vi "Periodic Tasks.vi"(8 "error in":errorcluster) -> ()   [LabVIEW 2013]
doc: "This VI runs in parallel to other tasks. It can contain as many user-defined periodic loops as you need. These can carry out PID or other sorts of timed response."
uses:
  <vilib>/Rock Robotics/WPI/Solenoid/WPI_SolenoidValue.ctl
  <vilib>/Rock Robotics/SystemInterfaces/Utilities/FPGA_UtilitiesLED Source.ctl
  <vilib>/Rock Robotics/SystemInterfaces/Utilities/FPGA_UtilitiesLED State.ctl
  <vilib>/Rock Robotics/WPI/Relay/WPI_RelayValue.ctl
  <vilib>/Rock Robotics/WPI/Compressor/WPI_CompressorGetSetRefNum.vi
  Robot Global Data.vi
  <vilib>/Rock Robotics/WPI/Joystick/WPI_JoystickGetSetRefNum.vi
  Global_firing.vi
  <vilib>/Rock Robotics/WPI/Solenoid/WPI_SolenoidSetEnum.vi
panel:
  in  "stop":bool
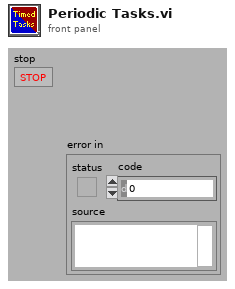
[diagram p1: front panel]
types:
  T1 = typedef "FPGA_UtilitiesLED State.ctl" = enum16{"Off", "On", "Toggle"}
  T2 = typedef "FPGA_UtilitiesLED Source.ctl" = enum16{"User LED", "FPGA LED"}
  T3 = typedef "WPI_CompressorDevRef.ctl" = cluster{"DevStatus":errorcluster, "DigitalInputDevRef":T4, "RelayDevRef":T7}
  T4 = typedef "WPI_DigitalInputDevRef.ctl" = cluster{"DevStatus":errorcluster, "DIO Channel":T5, "Digital Module":T6}
  T5 = typedef "FPGA_DIOChannel.ctl" = enum8{"DIO 1", "DIO 2", "DIO 3", "DIO 4", "DIO 5", "DIO 6", "DIO 7", "DIO 8", "DIO 9", "DIO 10", "DIO 11", "DIO 12", "DIO 13", "DIO 14", "Invalid"}
  T6 = typedef "FPGA_TypedefDigitalModule.ctl" = enum16{"Digital Module 1", "Digital Module 2"}
  T7 = typedef "WPI_RelayDevRef.ctl" = cluster{"DevStatus":errorcluster, "Relay Channel":T8, "Digital Module":T6, "Relay Direction":T9}
  T8 = typedef "FPGA_DIORelayChannel.ctl" = enum8{"Relay 1", "Relay 2", "Relay 3", "Relay 4", "Relay 5", "Relay 6", "Relay 7", "Relay 8", "Invalid"}
  T9 = typedef "WPI_RelayDirection.ctl" = enum16{"Both directions", "Forward only", "Reverse only"}
  T10 = typedef "WPI_SolenoidDevRef.ctl" = cluster{"DevStatus":errorcluster, "Solenoid Module":T11, "Forward Solenoid Channel":T12, "Reverse Solenoid Channel":T12}
  T11 = typedef "FPGA_TypedefSolenoidModule.ctl" = enum16{"Solenoid Module 1", "Solenoid Module 2"}
  T12 = typedef "WPI_SolenoidChannel.ctl" = enum8{"Solenoid 1", "Solenoid 2", "Solenoid 3", "Solenoid 4", "Solenoid 5", "Solenoid 6", "Solenoid 7", "Solenoid 8", "Invalid"}
  T13 = typedef "WPI_JoystickDevRef.ctl" = cluster{"Device":T14}
  T14 = typedef "WPI_JoystickDeviceEnum.ctl" = enum16{"USB 1", "USB 2", "USB 3", "USB 4", "Kinect 1", "Kinect 2"}
  T15 = typedef "WPI_MotorControlDeviceRef.ctl" = cluster{"DeviceStatus":errorcluster, "Type":enum16{"PWM", "CAN"}, "PWM":cluster{"Digital Module":T6, "PWM Channel":T16, "DeadBand":T17}, "CAN":cluster{"Device Number":u8, "Control Mode":T18, "Semaphore":T19, "Max Vout":dbl}, "Invert":bool, "TransformRef":T20, "InvTransformRef":T20}
  T16 = typedef "FPGA_DIOPWMChannel.ctl" = enum8{"PWM 1", "PWM 2", "PWM 3", "PWM 4", "PWM 5", "PWM 6", "PWM 7", "PWM 8", "PWM 9", "PWM 10", "Invalid"}
  T17 = typedef "WPI_PWMDeadband.ctl" = cluster{"Name":string, "maxPositivePwm":i32, "minPositivePwm":i32, "centerPwm":i32, "maxNegativePwm":i32, "minNegativePwm":i32, "angularRange":u16}
  T18 = typedef "WPI_CANJaguar_ControlMode.ctl" = enum8{"Percent VBus", "Current", "Speed", "Position", "Voltage"}
  T19 = typedef "Semaphore RefNum" = refnum<k1>
  T20 = typedef "WPI_PWMTransform_ConPane.ctl" = refnum<vi>
  T21 = cluster{"JoystickDevRef":T13, "JoystickDevRef":T13, "SolenoidDevRef":T10, "SolenoidDevRef":T10, "SolenoidDevRef":T10, "SolenoidDevRef":T10, "RelayDevRef":T7, "MotorControlDevRef":T15}
  T22 = typedef "WPI_SolenoidValue.ctl" = enum16{"Off", "On", "Forward", "Reverse"}
  T23 = typedef "WPI_RelayValue.ctl" = enum16{"Off", "On", "Forward", "Reverse"}
  T24 = typedef "WPI_JoystickButtonState.ctl" = cluster{"Button 1":bool, "Button 2":bool, "Button 3":bool, "Button 4":bool, "Button 5":bool, "Button 6":bool, "Button 7":bool, "Button 8":bool, "Button 9":bool, "Button 10":bool, "Button 11":bool, "Button 12":bool}
  T25 = cluster{"axis 1 (x)":dbl, "axis 2 (y)":dbl, "axis 3 (throttle)":dbl, "axis 4":dbl, "axis 5":dbl, "axis 6":dbl}
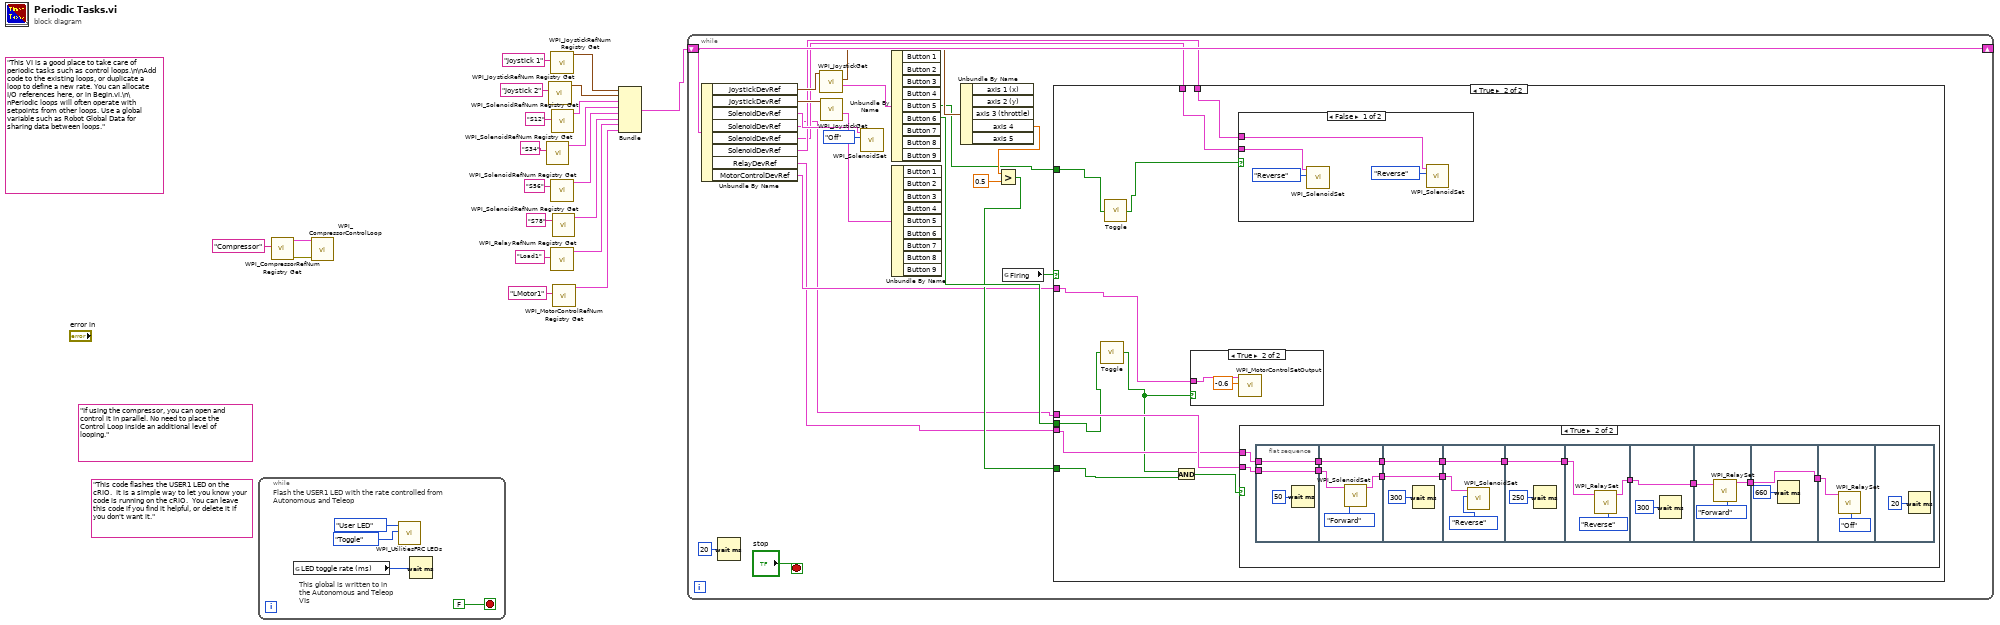
[diagram p0: block diagram]
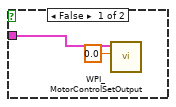
[diagram p2: hidden frame]
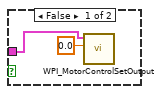
[diagram p3: hidden frame]
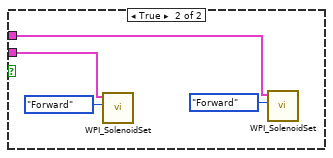
[diagram p4: hidden frame]
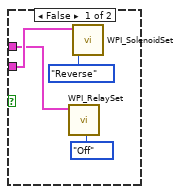
[diagram p5: hidden frame]
diagram:
  (unwired) "If using the compressor, you can open and control it in parallel. No need to place the Control Loop inside an additional level of looping."
  (unwired) "This code flashes the USER1 LED on the cRIO.  It is a simple way to let you know your code is running on the cRIO.  You can leave this code if you find it helpful, or delete it if you don't want it."
  (unwired) "This VI is a good place to take care of periodic tasks such as control loops.\n\nAdd code to the existing loops, or duplicate a loop to define a new rate. You can allocate I/O references here, or in Begin.vi.\n\nPeriodic loops will often operate with setpoints from other loops. Use a global variable such as Robot Global Data for sharing data between loops."
  n1 = while {
    stop <- FALSE stop-if-true
    # "This global is written to in the Autonomous and Teleop VIs"
    # "Flash the USER1 LED with the rate controlled from Autonomous and Teleop"
    n2 = global read "Robot Global Data.vi" "LED toggle rate (ms)"() -> (w21:u32)
    n3 = call <vilib>:"WPI_UtilitiesFRC LEDs.vi"("State"=FPGA_UtilitiesLED_State."Toggle", "LED Type"=FPGA_UtilitiesLED_Source."User LED") -> ()  [unwired: 1 in, 9 out]
    n4 = Wait (ms)(milliseconds to wait=w21) -> ()  [unwired: 1 out]
  }
  n5 = call <vilib>:"WPI_CompressorRefNum Registry Get.vi"("refnum name"="Compressor") -> ("error out"=w1:errorcluster, "CompressorDevRef"=w2:T3)  [unwired: 9 in]
  n6 = call <vilib>:"WPI_CompressorControlLoop.vi"("error in (no error)"=w1, "CompressorDevRef"=w2) -> ()  [unwired: 10 in]
  n7 = call <vilib>:"WPI_SolenoidRefNum Registry Get.vi"("refnum name"="S34") -> ("SolenoidDevRef"=w9:T10)  [unwired: 9 in, 1 out]
  n8 = call <vilib>:"WPI_JoystickRefNum Registry Get.vi"("refnum name"="Joystick 2") -> ("JoystickDevRef"=w11:T13)  [unwired: 9 in, 1 out]
  n9 = call <vilib>:"WPI_JoystickRefNum Registry Get.vi"("refnum name"="Joystick 1") -> ("JoystickDevRef"=w12:T13)  [unwired: 9 in, 1 out]
  n10 = call <vilib>:"WPI_SolenoidRefNum Registry Get.vi"("refnum name"="S56") -> ("SolenoidDevRef"=w8:T10)  [unwired: 9 in, 1 out]
  n11 = call <vilib>:"WPI_RelayRefNum Registry Get.vi"("refnum name"="Load1") -> ("RelayDevRef"=w6:T7)  [unwired: 9 in, 1 out]
  n12 = call <vilib>:"WPI_SolenoidRefNum Registry Get.vi"("refnum name"="S12") -> ("SolenoidDevRef"=w10:T10)  [unwired: 9 in, 1 out]
  n13 = call <vilib>:"WPI_SolenoidRefNum Registry Get.vi"("refnum name"="S78") -> ("SolenoidDevRef"=w7:T10)  [unwired: 9 in, 1 out]
  n14 = call <vilib>:"WPI_MotorControlRefNum Registry Get.vi"("refnum name"="LMotor1") -> ("MotorControlDevRef"=w5:T15)  [unwired: 9 in, 1 out]
  n15 = Bundle("JoystickDevRef"=w12, "JoystickDevRef"=w11, "SolenoidDevRef"=w10, "SolenoidDevRef"=w9, "SolenoidDevRef"=w8, "SolenoidDevRef"=w7, "RelayDevRef"=w6, "MotorControlDevRef"=w5) -> (w4:T21)  [unwired: 1 in]
  n16 = while {
    shift-right: [w43] -> _
    shift-left: w4 -> [w43]
    stop <- "stop" stop-if-true
    n17 = Unbundle By Name(w43) -> ("JoystickDevRef"=w40:T13, "JoystickDevRef"=w41:T13, "SolenoidDevRef"=w36:T10, "SolenoidDevRef"=w26:T10, "SolenoidDevRef"=w28:T10, "SolenoidDevRef"=w29:T10, "RelayDevRef"=w25:T7, "MotorControlDevRef"=w27:T15)
    n18 = Wait (ms)(milliseconds to wait=u32 20) -> ()  [unwired: 1 out]
    n19 = call <vilib>:"WPI_JoystickGet.vi"("JoystickDevRef"=w40) -> ("Buttons"=w39:T24, "Axes"=w34:T25)  [unwired: 4 in, 1 out]
    n20 = call <vilib>:"WPI_JoystickGet.vi"("JoystickDevRef"=w41) -> ("Buttons"=w38:T24)  [unwired: 4 in, 2 out]
    n21 = call-poly <vilib>:"WPI_SolenoidSet.vi"("Value"=WPI_SolenoidValue."Off", "SolenoidDevRef"=w36) -> ()  [unwired: 8 in, 2 out]
    n22 = Unbundle By Name(w39) -> ("Button 5"=w30:bool, "Button 6"=w35:bool)  [unwired: 7 out]
    n23 = Unbundle By Name(w38) -> ()  [unwired: 9 out]
    n24 = Unbundle By Name(w34) -> ("axis 4"=w32:dbl)  [unwired: 4 out]
    n25 = Greater?(x=w32, y=0.5) -> (0:w31:bool)
    n26 = global read "Global_firing.vi" "Firing"() -> (w37:bool)
    n27 = case shown="True" w37 {
      tunnel: w35 -> [_ w49]
      tunnel: w31 -> [_ w54]
      tunnel: w30 -> [_ w51]
      tunnel: w29 -> [_ w56]
      tunnel: w28 -> [_ w57]
      tunnel: w27 -> [w46 w55]
      tunnel: w26 -> [_ w53]
      tunnel: w25 -> [_ w52]
      frame False {
        n28 = call <vilib>:"WPI_MotorControlSetOutput.vi"("Output"=0.0, "MotorControlDevRef"=w46) -> ()  [unwired: 7 in, 3 out]
      }
      frame True {
        n29 = call "Toggle.vi"("Input"=w49) -> ("Output"=w48:bool)
        n30 = call "Toggle.vi"("Input"=w51) -> ("Output"=w50:bool)
        n31 = And(x=w48, y=w54) -> (x .and. y?=w58:bool)
        n32 = case shown="True" w48 {
          tunnel: w55 -> [w59 w62]
          frame False {
            n33 = call <vilib>:"WPI_MotorControlSetOutput.vi"("Output"=0.0, "MotorControlDevRef"=w59) -> ()  [unwired: 7 in, 3 out]
          }
          frame True {
            n34 = call <vilib>:"WPI_MotorControlSetOutput.vi"("Output"=-0.6, "MotorControlDevRef"=w62) -> ()  [unwired: 7 in, 3 out]
          }
        }
        n35 = case shown="False" w50 {
          tunnel: w57 -> [w64 w69]
          tunnel: w56 -> [w63 w68]
          frame False {
            n36 = call-poly <vilib>:"WPI_SolenoidSet.vi"("Value"=WPI_SolenoidValue."Reverse", "SolenoidDevRef"=w64) -> ()  [unwired: 8 in, 2 out]
            n37 = call-poly <vilib>:"WPI_SolenoidSet.vi"("Value"=WPI_SolenoidValue."Reverse", "SolenoidDevRef"=w63) -> ()  [unwired: 8 in, 2 out]
          }
          frame True {
            n38 = call-poly <vilib>:"WPI_SolenoidSet.vi"("Value"=WPI_SolenoidValue."Forward", "SolenoidDevRef"=w69) -> ()  [unwired: 8 in, 2 out]
            n39 = call-poly <vilib>:"WPI_SolenoidSet.vi"("Value"=WPI_SolenoidValue."Forward", "SolenoidDevRef"=w68) -> ()  [unwired: 8 in, 2 out]
          }
        }
        n40 = case shown="True" w58 {
          tunnel: w53 -> [w72 w88]
          tunnel: w52 -> [w71 w84]
          frame False {
            n41 = call <vilib>:"WPI_RelaySet.vi"("RelayValue"=WPI_RelayValue."Off", "RelayDevRef"=w71) -> ()  [unwired: 8 in, 2 out]
            n42 = call-poly <vilib>:"WPI_SolenoidSet.vi"("Value"=WPI_SolenoidValue."Reverse", "SolenoidDevRef"=w72) -> ()  [unwired: 8 in, 2 out]
          }
          frame True {
            n43 = flat-sequence {
              tunnel: w88 -> [w90]
              tunnel: [w90] -> w87
              tunnel: w84 -> [w89]
              tunnel: [w89] -> w83
              tunnel: w87 -> [w94]
              tunnel: [w93] -> w86
              tunnel: w83 -> [w92]
              tunnel: [w92] -> w82
              tunnel: w86 -> [w97]
              tunnel: [w97] -> w85
              tunnel: w82 -> [w96]
              tunnel: [w96] -> w81
              tunnel: w85 -> [w100]
              tunnel: w81 -> [w99]
              tunnel: [w99] -> w80
              tunnel: w80 -> [w102]
              tunnel: [w102] -> w79
              tunnel: w79 -> [w105]
              tunnel: [w104] -> w78
              tunnel: w78 -> [w107]
              tunnel: [w107] -> w77
              tunnel: w77 -> [w110]
              tunnel: [w109] -> w76
              tunnel: w76 -> [w112]
              tunnel: [w112] -> w75
              tunnel: w75 -> [w114]
              frame #0 {
                n44 = Wait (ms)(milliseconds to wait=u32 50) -> ()  [unwired: 1 out]
              }
              frame #1 {
                n45 = call-poly <vilib>:"WPI_SolenoidSet.vi"("Value"=WPI_SolenoidValue."Forward", "SolenoidDevRef"=w94) -> ("SolenoidDevRef"=w93:T10)  [unwired: 8 in, 1 out]
              }
              frame #2 {
                n46 = Wait (ms)(milliseconds to wait=u32 300) -> ()  [unwired: 1 out]
              }
              frame #3 {
                n47 = call-poly <vilib>:"WPI_SolenoidSet.vi"("Value"=WPI_SolenoidValue."Reverse", "SolenoidDevRef"=w100) -> ()  [unwired: 8 in, 2 out]
              }
              frame #4 {
                n48 = Wait (ms)(milliseconds to wait=u32 250) -> ()  [unwired: 1 out]
              }
              frame #5 {
                n49 = call <vilib>:"WPI_RelaySet.vi"("RelayValue"=WPI_RelayValue."Reverse", "RelayDevRef"=w105) -> ("RelayDevRef"=w104:T7)  [unwired: 8 in, 1 out]
              }
              frame #6 {
                n50 = Wait (ms)(milliseconds to wait=u32 300) -> ()  [unwired: 1 out]
              }
              frame #7 {
                n51 = call <vilib>:"WPI_RelaySet.vi"("RelayValue"=WPI_RelayValue."Forward", "RelayDevRef"=w110) -> ("RelayDevRef"=w109:T7)  [unwired: 8 in, 1 out]
              }
              frame #8 {
                n52 = Wait (ms)(milliseconds to wait=u32 660) -> ()  [unwired: 1 out]
              }
              frame #9 {
                n53 = call <vilib>:"WPI_RelaySet.vi"("RelayValue"=WPI_RelayValue."Off", "RelayDevRef"=w114) -> ()  [unwired: 8 in, 2 out]
              }
              frame #10 {
                n54 = Wait (ms)(milliseconds to wait=u32 20) -> ()  [unwired: 1 out]
              }
            }
          }
        }
      }
    }
  }
